vi "Data Array 만들기.vi"() -> ()   [LabVIEW 2019]
panel:
  out "Numeric":dbl
  out "Waveform Graph":dbl[](graph)
  out "Array":dbl[](array[numeric])
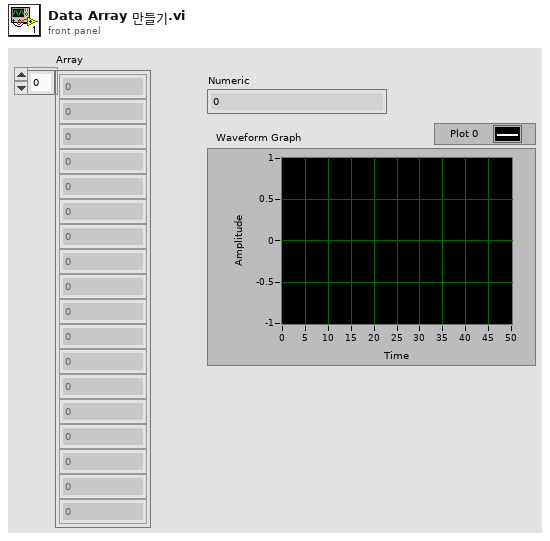
[diagram p1: front panel]
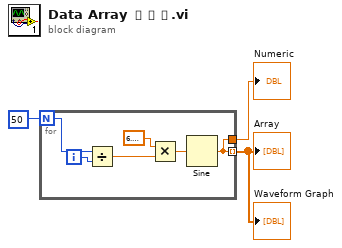
[diagram p0: block diagram]
diagram:
  n1 = for {
    N: 50 -> [w6]
    tunnel: [w8] -> w1 mode=indexing
    tunnel: [w8] -> w2
    i -> [w5]
    n2 = Divide(x=w6, y=w5) -> (x/y=w7:dbl)
    n3 = Multiply(x=6.283185307179586, y=w7) -> (x*y=w9:dbl)
    n4 = Sine(x=w9) -> (sin(x)=w8:dbl)
  }
  "Array" <- w1
  "Waveform Graph" <- w1
  "Numeric" <- w2
